vi "STP_Client.vi"(8 "error in (no error)":errorcluster, 9 "data to send":string, 10 "Command":T1, 11 "address":string) -> (0 "error out":errorcluster, 1 "data received from server":string)   [LabVIEW 2020]
uses:
  <vilib>/NI/STM/SubVIs/MetaDataElement.ctl
  Typedefs/Remote-SMO-Commands-Enum.ctl
  <vilib>/NI/STM/TCP/TCP Read Options.ctl
  <vilib>/NI/STM/TCP/Read Meta Data (TCP Ref).vi
  <vilib>/NI/STM/TCP/Get Connection Reference (TCP).vi
  <vilib>/NI/STM/TCP/Read Meta Data (TCP Clst).vi
  <vilib>/NI/STM/TCP/Write Message (TCP).vi
  <vilib>/NI/STM/TCP/Read Message (TCP).vi
  <userlib>/_OpenG.lib/error/error.llb/Filter Error Codes (Array)__ogtk.vi
  <vilib>/NI/STM/NI STM.lvlib
  RemoteControl.lvclass
panel:
  out "since last call ms":u32
  out "duration ms":u32
  out "available commands = enum?":bool
  out "meta data (available commands)":T2[](array[typedef])
  # "CLIENT (API)"
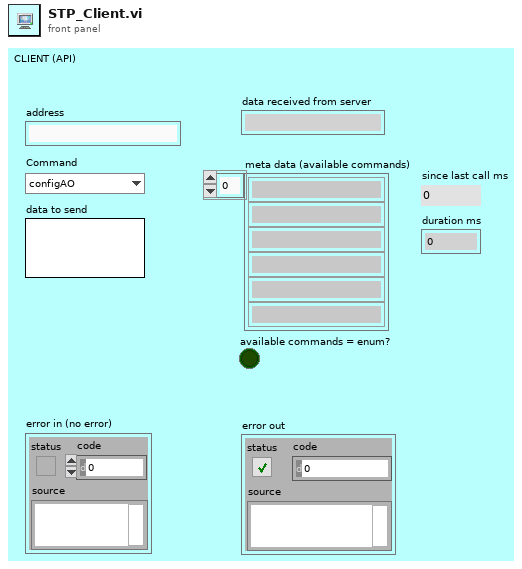
[diagram p1: front panel]
types:
  T1 = typedef "RemoteControl.lvclass/Remote-SMO-Commands-Enum.ctl" = enum16{"configAO", "configREF", "configIVmode", "configRemote", "configReset", "assertTrigger", "getAO", "getAI", "getResults", "getTrigger", "getIVmode", "getAOconfig", "getREFconfig", "ACK", "UNK", "CLOSE"}
  T2 = typedef "NI STM.lvlib/MetaDataElement.ctl" = string
  T3 = typedef "NI STM.lvlib/TCP Read Options.ctl" = cluster{"ignore timeout error":bool, "timeout ms (1000)":i32}
  T4 = typedef "NI STM.lvlib/TCP Connection Info.ctl" = cluster{"connection ID":refnum<k5>, "meta data":T2[]}
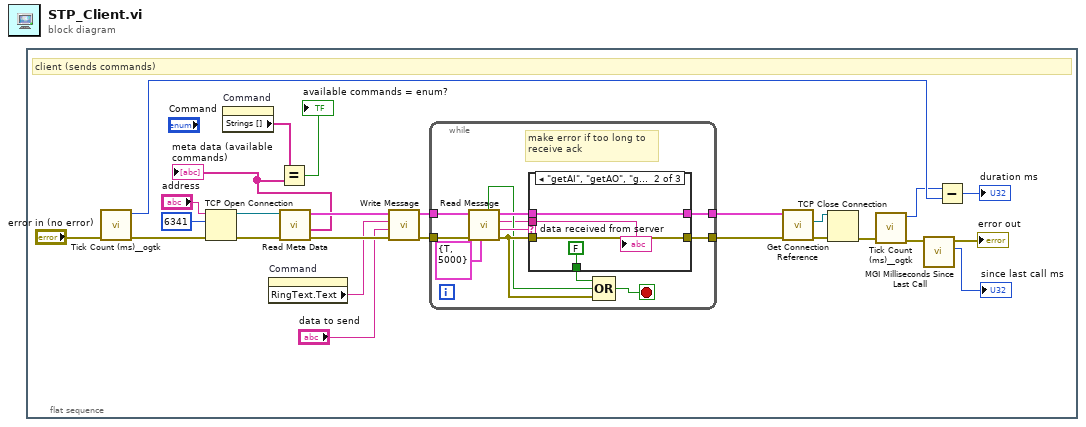
[diagram p0: block diagram]
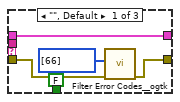
[diagram p2: hidden frame]
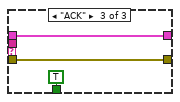
[diagram p3: hidden frame]
diagram:
  n1 = flat-sequence {
    frame #0 {
      # "client (sends commands)"
      n2 = call <userlib>:"Tick Count (ms)__ogtk.vi"("error in (no error)"="error in (no error)") -> ("error out"=w13:errorcluster, "millisecond timer value"=w4:u32)  [unwired: 9 in]
      n3 = TCP Open Connection(address="address", remote port or service name=u16 6341, error in (no error)=w13) -> (connection ID=w21:refnum<k5>, error out=w22:errorcluster)  [unwired: 2 in]
      n4 = property on="Command" class="Enum (strict)"() -> ("Strings []"=w20:string[])  [unwired: 2 in, 2 out]
      n5 = property on="Command" class="Enum (strict)"() -> ("RingText.Text"=w12:string)  [unwired: 2 in, 2 out]
      n6 = call-poly <vilib>:"Read Meta Data.vi"("error in"=w22, "connection ID"=w21) -> ("error out"=w25:errorcluster, "meta data"=w17:T2[], "connection info out"=w26:T4)  [unwired: 7 in]
      "meta data (available commands)" <- w17
      n7 = Equal?(x=w20, y=w17) -> (x = y?=→"available commands = enum?":bool)
      n8 = call-poly <vilib>:"Write Message.vi"("error in"=w25, "data"="data to send", "name"=w12, "connection info in"=w26) -> ("error out"=w24:errorcluster, "connection info out"=w23:T4)  [unwired: 6 in]
      n9 = while {
        tunnel: w24 -> [w38]
        tunnel: w23 -> [w37]
        tunnel: [w35] -> w2
        tunnel: [w33] -> w1
        stop <- w32 stop-if-true
        # "make error if too long to\nreceive ack"
        n10 = call-poly <vilib>:"Read Message.vi"("options"=T3 {"ignore timeout error"=TRUE, "timeout ms (1000)"=5000}, "error in"=w38, "connection info in"=w37) -> ("error out"=w31:errorcluster, "name"=w36:T2, "data string"=w29:string, "connection info out"=w34:T4, "timed out?"=w30:bool)  [unwired: 1 in, 3 out]
        n11 = case shown="\"getAI\", \"getAO\", \"getAOconfig\", \"getIVmode\", \"getREFconfig\", \"getResults\", \"getTrigger\"" w36 {
          tunnel: w31 -> [w40 w47 w49]
          tunnel: [w42 w47 w49] -> w35
          tunnel: w34 -> [w43 w46 w50]
          tunnel: [w43 w46 w50] -> w33
          tunnel: w29 -> [_ w45 _]
          tunnel: [FALSE ("value") FALSE ("value") TRUE ("value")] -> w27
          frame "", Default {
            n12 = call-poly <userlib>:"Filter Error Codes__ogtk.vi"("Error In"=w40, "Error Codes to Filter"=i32[] [66]) -> ("Error Out"=w42:errorcluster)  [unwired: 7 in, 2 out]
          }
          frame "getAI", "getAO", "getAOconfig", "getIVmode", "getREFconfig", "getResults", "getTrigger" {
            "data received from server" <- w45
          }
          frame "ACK" {
          }
        }
        n13 = Compound Arithmetic op=OR(w27, w30, w31) -> (w32:bool)
      }
      n14 = call-poly <vilib>:"Get Connection Reference.vi"("error in"=w2, "connection info in"=w1) -> ("error out"=w15:errorcluster, "connection ID out"=w14:refnum<k5>)  [unwired: 7 in, 1 out]
      n15 = TCP Close Connection(connection ID=w14, error in (no error)=w15) -> (error out=w11:errorcluster)  [unwired: 1 in, 1 out]
      n16 = call <userlib>:"Tick Count (ms)__ogtk.vi"("error in (no error)"=w11) -> ("error out"=w9:errorcluster, "millisecond timer value"=w3:u32)  [unwired: 9 in]
      n17 = call <userlib>:"MGI Milliseconds Since Last Call.vi"("Error In"=w9) -> ("ms"=→"since last call ms":u32, "Error Out"=→"error out":errorcluster)  [unwired: 5 in]
      n18 = Subtract(x=w3, y=w4) -> (x-y=→"duration ms":u32)
    }
  }
